vi "CreatePitchValuesINI.vi"(2 "error in (no error)":errorcluster, 3 "configuration file path":path) -> (0 "error out":errorcluster, 1 "file path":path)   [LabVIEW 2012]
uses:
  <vilib>/Utility/config.llb/Write Key (Double).vi
  <vilib>/Utility/config.llb/NI_LVConfig.lvlib
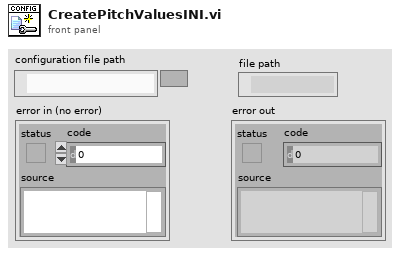
[diagram p1: front panel]
types:
  T1 = typedef "NI_LVConfig.lvlib/Config Data RefNum.ctl" = refnum<k1>
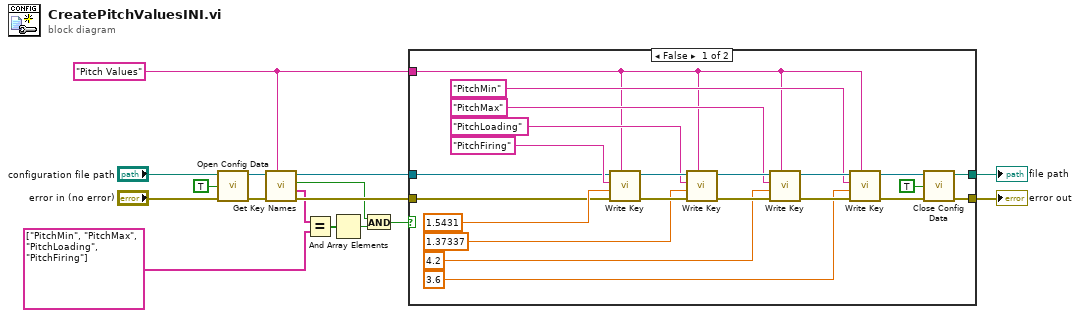
[diagram p0: block diagram]
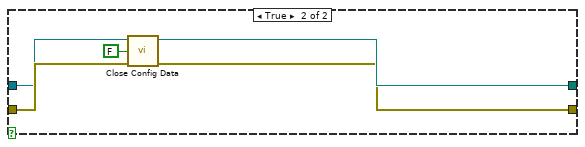
[diagram p2: hidden frame]
diagram:
  w13 = "Pitch Values"
  n1 = call <vilib>:"Open Config Data.vi"("error in (no error)"="error in (no error)", "create file if necessary (T)"=TRUE, "configuration file path"="configuration file path") -> ("error out"=w14:errorcluster, "refnum"=w15:T1)  [unwired: 6 in, 1 out]
  n2 = call <vilib>:"Get Key Names.vi"("section"=w13, "error in (no error)"=w14, "refnum"=w15) -> ("error out"=w11:errorcluster, "key names"=w10:string[], "section exists?"=w6:bool, "refnum out"=w12:T1)  [unwired: 5 in]
  n3 = Equal?(x=w10, y=string[] ["PitchMin", "PitchMax", "PitchLoading", "PitchFiring"]) -> (x = y?=w8:bool[])
  n4 = And Array Elements(Boolean array=w8) -> (logical AND=w7:bool)
  n5 = And(x=w6, y=w7) -> (x .and. y?=w5:bool)
  n6 = case shown="False" w5 {
    tunnel: w13 -> [w25 _]
    tunnel: w12 -> [w21 w39]
    tunnel: w11 -> [w20 w40]
    tunnel: [w24 w42] -> w2
    tunnel: [w23 w41] -> w1
    frame False {
      n7 = call-poly <vilib>:"Write Key.vi"("section"=w25, "error in (no error)"=w20, "value"=1.5431, "key"="PitchFiring", "refnum"=w21) -> ("error out"=w35:errorcluster, "refnum out"=w36:T1)  [unwired: 4 in, 1 out]
      n8 = call-poly <vilib>:"Write Key.vi"("section"=w25, "error in (no error)"=w35, "value"=1.37337, "key"="PitchLoading", "refnum"=w36) -> ("error out"=w38:errorcluster, "refnum out"=w30:T1)  [unwired: 4 in, 1 out]
      n9 = call-poly <vilib>:"Write Key.vi"("section"=w25, "error in (no error)"=w38, "value"=4.2, "key"="PitchMax", "refnum"=w30) -> ("error out"=w33:errorcluster, "refnum out"=w34:T1)  [unwired: 4 in, 1 out]
      n10 = call-poly <vilib>:"Write Key.vi"("section"=w25, "error in (no error)"=w33, "value"=3.6, "key"="PitchMin", "refnum"=w34) -> ("error out"=w32:errorcluster, "refnum out"=w31:T1)  [unwired: 4 in, 1 out]
      n11 = call <vilib>:"Close Config Data.vi"("error in (no error)"=w32, "write file if changed (T)"=TRUE, "refnum"=w31) -> ("error out"=w23:errorcluster, "file path"=w24:path)  [unwired: 7 in]
    }
    frame True {
      n12 = call <vilib>:"Close Config Data.vi"("error in (no error)"=w40, "write file if changed (T)"=FALSE, "refnum"=w39) -> ("error out"=w41:errorcluster, "file path"=w42:path)  [unwired: 7 in]
    }
  }
  "file path" <- w2
  "error out" <- w1
